vi "inverse_josephus.vi"() -> ()   [LabVIEW 2019]
panel:
  out "Start at":dbl
  in  "Last":dbl
  in  "m":dbl
  in  "N":dbl
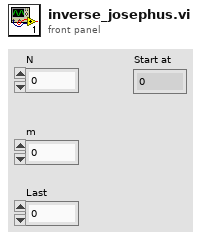
[diagram p1: front panel]
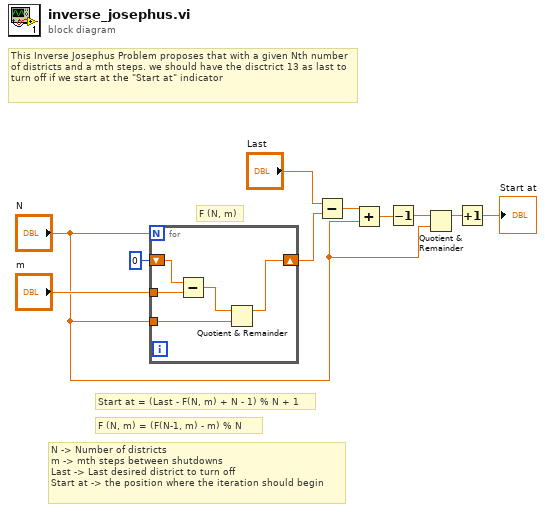
[diagram p0: block diagram]
diagram:
  # "F (N, m) = (F(N-1, m) - m) % N"
  # "F (N, m)"
  # "Start at = (Last - F(N, m) + N - 1) % N + 1"
  # "N -> Number of districts\nm -> mth steps between shutdowns\nLast -> Last desired district to turn off\nStart at -> the position where the iteration should begin"
  # "This Inverse Josephus Problem proposes that with a given Nth number of districts and a mth steps. we should have the disctrict 13 as last to turn off if we start at the \"Start at\" indicator"
  n1 = for {
    N: "N" -> [_]
    shift-right: [w11] -> w7
    shift-left: 0 -> [w12]
    tunnel: "N" -> [w14]
    tunnel: "m" -> [w13]
    n2 = Subtract(x=w12, y=w13) -> (x-y=w15:dbl)
    n3 = Quotient & Remainder(x=w15, y=w14) -> (x-y*floor(x/y)=w11:dbl)  [unwired: 1 out]
  }
  n4 = Subtract(x="Last", y=w7) -> (x-y=w6:dbl)
  n5 = Add(x=w6, y="N") -> (x+y=w5:dbl)
  n6 = Decrement(x=w5) -> (x-1=w4:dbl)
  n7 = Quotient & Remainder(x=w4, y="N") -> (x-y*floor(x/y)=w3:dbl)  [unwired: 1 out]
  n8 = Increment(x=w3) -> (x+1=→"Start at":dbl)
